vi "RT TEST.vi"() -> ()   [LabVIEW 2017]
uses:
  <vilib>/Platform/TimedLoop/XDataNode/timing_clust.ctl
  <vilib>/Platform/TimedLoop/XDataNode/nitl_modes.ctl
  <vilib>/Platform/TimedLoop/XDataNode/wakeup.ctl
  <vilib>/myRIO/Common/Instrument Driver Framework/myRIO v1.0/UART/vis/myRIO v1.0 Close UART.vi
  <vilib>/FPGAPlugInAG/myRIO-1900/niLvFpga_Open_myRIO-1900.vi
  <vilib>/rvi/interface/common/dynamic/niFpgaDynamicAddResources.vi
  <vilib>/myRIO/Common/Instrument Driver Framework/Utilities/vis/FPGA Ref Manager.vi
  <vilib>/Utility/error.llb/Error Cluster From Error Code.vi
  <vilib>/myRIO/Common/Instrument Driver Framework/Utilities/vis/Ref Counter.vi
  <vilib>/FPGAPlugInAG/Dynamic/niLvFpga_Close_Dynamic.vi
  <vilib>/myRIO/Common/Instrument Driver Framework/myRIO v1.0/myRIO v1.0 Reset FPGA.vi
  <vilib>/myRIO/Common/Instrument Driver Framework/myRIO v1.0/IRQ/vis/myRIO v1.0 IRQ Info FGV.vi
  <vilib>/myRIO/Common/Instrument Driver Framework/myRIO v1.0/IRQ/vis/myRIO v1.0 Timer IRQ Info FGV.vi
  <vilib>/myRIO/Common/Instrument Driver Framework/myRIO v1.0/IRQ/vis/myRIO v1.0 ISR Agent.vi
  <vilib>/rvi/interface/nirviOpenFPGA/nirviOpenFPGA.xnode
  <vilib>/Platform/TimedLoop/XDataNode/XDataNode.xnode
  <vilib>/rvi/interface/nirviCloseFPGA/nirviCloseFPGA.xnode
  <vilib>/Platform/TimedLoop/XDataNode/XDNodeRunTimeDep.lvlib
  <vilib>/myRIO/Instrument Drivers/Utilities/Utilities.lvlib
panel:
  in  "停止":bool
  in  "频率":u16=20000
  out "ENC":i32[](array[numeric])=[1, 0, -1, -1, 1, 0]
  in  "Reset ENC":bool
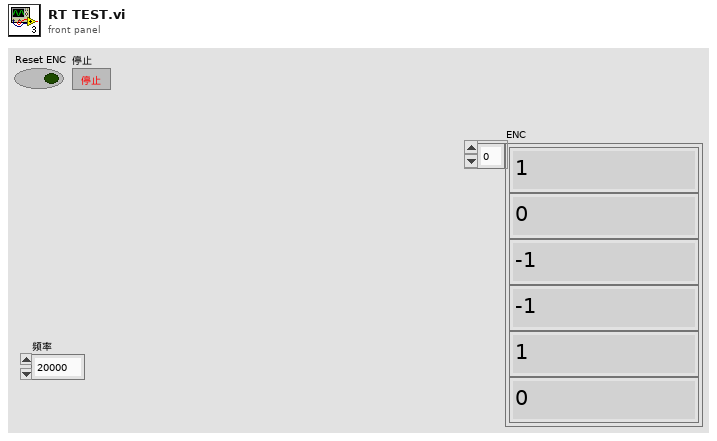
[diagram p1: front panel]
types:
  T1 = typedef "XDNodeRunTimeDep.lvlib/timing_clust.ctl" = cluster{"Expected End [f-1]":u64, "Actual End [f-1]":u64, "Finished Late? [f-1]":bool, "Expected End [i-1]":u64, "Actual End [i-1]":u64, "Finished Late? [i-1]":bool, "Expected Start [i]":u64, "Actual Start [i]":u64, "Expected Start [f]":u64, "Actual Start [f]":u64, "Source Name":string, "Structure Name":string, "Period":i64, "Deadline":i64, "Offset":i64, "Start":i64, "Priority":i32, "Timeout":i32, "Mode":T2, "Wakeup Reason":T3, "Error":errorcluster, "Source Type":string, "Secondary Source Type":string, "Global End Time":u64, "Global Start Time":u64, "Frame Duration":u64, "Iteration Duration":u64, "Assigned CPU":i32, "I/O Scan Engine Mode":u32}
  T2 = typedef "XDNodeRunTimeDep.lvlib/nitl_modes.ctl" = enum32{"No Change", "Process missed periods, maintain original phase", "Discard missed periods, maintain original phase", "Process missed periods, ignore original phase", "Discard missed periods, ignore original phase"}
  T3 = typedef "XDNodeRunTimeDep.lvlib/wakeup.ctl" = enum32{"Normal", "Aborted", "Asynchronous wakeup", "Timing source error", "Timed loop error", "Timeout"}
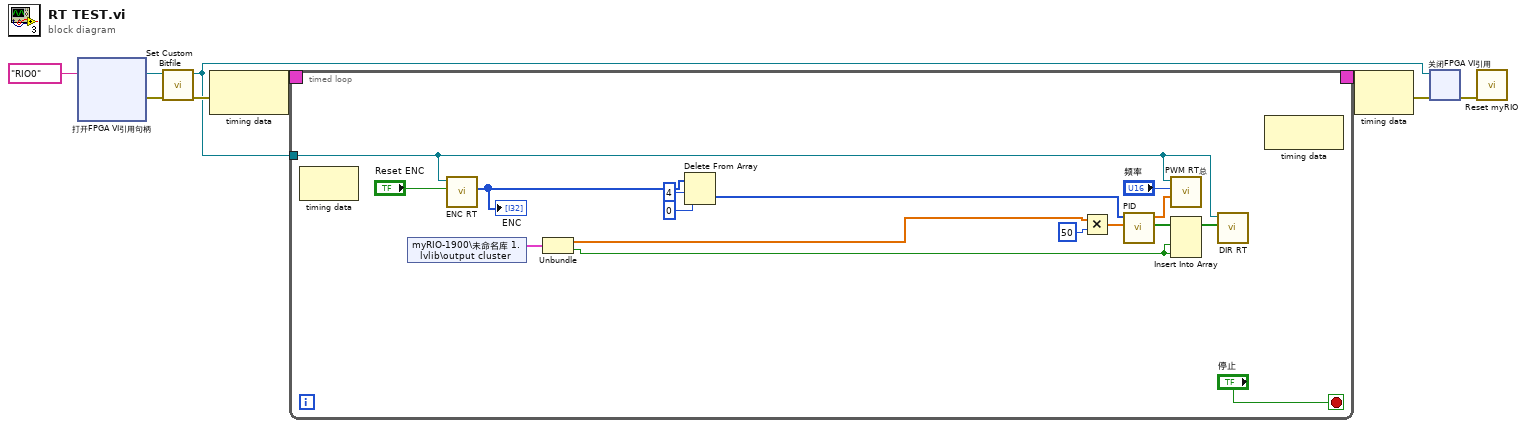
[diagram p0: block diagram]
diagram:
  n1 = xnode "打开FPGA VI引用句柄"("资源名称"=tag "RIO0") -> ("FPGA VI引用输出"=w7:refnum<k20>, "错误输出"=w6:errorcluster)  [unwired: 1 in]
  n2 = call <vilib>:"Set Custom Bitfile.vi"("error in (no error)"=w6, "Custom FPGA Reference In"=w7) -> ("error out"=w4:errorcluster, "Custom FPGA Reference Out"=w2:refnum<k20>)  [unwired: 8 in]
  n3 = node-c288(w4) -> (w9:T1)
  n4 = timed-loop {
    timing: w9 -> [_]
    timing-out: [_] -> w8
    tunnel: w2 -> [w24]
    stop <- "停止" stop-if-true
    n5 = node-c288() -> ()  [unwired: 1 in, 1 out]
    n6 = shared-variable "myRIO-1900\\未命名库 1.lvlib\\output cluster"() -> (w19:cluster{dbl[], bool})  [unwired: 1 in, 1 out]
    n7 = call "ENC RT.vi"("Reset ENC"="Reset ENC", "Custom FPGA Reference Out"=w24) -> ("ENC"=w13:i32[])  [unwired: 7 in, 2 out]
    "ENC" <- w13
    n8 = Unbundle(w19) -> (w16:dbl[], w14:bool)
    n9 = Delete From Array(array=w13, length=4 ("长度"), index=0 ("索引")) -> (deleted portion=w10:i32[])  [unwired: 1 out]
    n10 = Multiply(x=w16, y=50) -> (x*y=w15:dbl[])
    n11 = call "PID.vi"("SET"=w15, "ENC"=w10) -> ("DIR"=w21:bool[], "PWM"=w17:dbl[])  [unwired: 8 in]
    n12 = call "PWM RT总.vi"("PWM"=w17, "频率"="频率", "Custom FPGA Reference Out"=w24) -> ()  [unwired: 7 in, 2 out]
    n13 = Insert Into Array(array=w21, new element #1=w14, new element #2=w14) -> (w20:bool[])  [unwired: 1 in]
    n14 = call "DIR RT.vi"("DIR"=w20, "Custom FPGA Reference Out"=w24) -> ()  [unwired: 8 in, 2 out]
    n15 = node-c288() -> ()  [unwired: 1 in, 1 out]
  }
  n16 = node-c288(w8) -> (w3:errorcluster)
  n17 = xnode "关闭FPGA VI引用"("FPGA VI引用输入"=w2, "错误输入"=w3) -> ("错误输出"=w5:errorcluster)
  n18 = call <vilib>:"Reset myRIO.vi"("error in (no error)"=w5) -> ()  [unwired: 10 in, 1 out]
